vi "Untitled 1.vi"() -> ()   [LabVIEW 2016]
uses:
  DISGradingMachine/MotionPackage/MotionPack/DISActFunc.ctl
panel:
  out "appended array 2":T1[](array[typedef])
  in  "appended array":T1[](array[typedef])
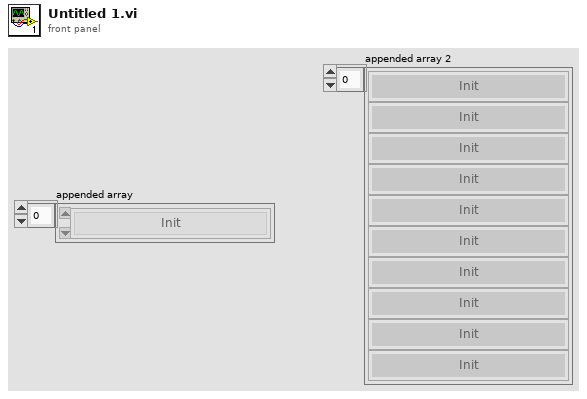
[diagram p1: front panel]
types:
  T1 = typedef "DISActFunc.ctl" = enum16{"Init", "X1 Go To Vibration Station", "X2 Go To DetectPos", "Z1 Go To Upper", "Z2 Go PickingPos(Par_UnitHeight)", "Y1_Go_To_Loose_Unit", "Y2_Go_To_Unit_Wide(Par_UnitWide)", "R Station1", "R Station2", "R Station3", "R Station4", "R Station5", "R Station6", "R Station7", "Vibration On", "Vibration Off", "1_Vacuum_On", "2_Vacuum_On", "3_Vacuum_On", "4_Vacuum_On", "5_Vacuum_On", "6_Vacuum_On", "1_Check_Vacuum", "2_Check_Vacuum", "3_Check_Vacuum", "4_Check_Vacuum", "5_Check_Vacuum", "6_Check_Vacuum", "Vacuum_All_Off", "Vacuum_All_Relief", "Pick6_Vacuum_Relief", "Cylinder_Fix_Unit", "Cylinder_UnFix_Unit", "Level_Probe_Cylinder_Extends", "Level_Probe_Cylinder_Retract", "Vertical_Probe_Cylinder_Extends", "Vertical_Probe_Cylinder_Retract", "Feeder_Inposition_On?"}
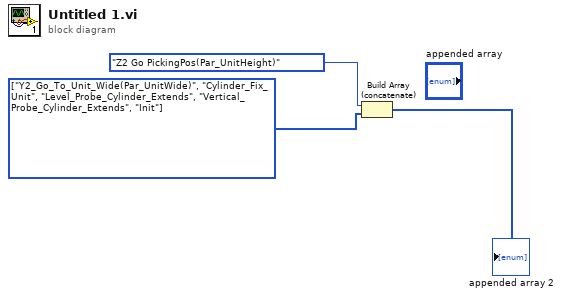
[diagram p0: block diagram]
diagram:
  w3 = T1[] [enum."Y2_Go_To_Unit_Wide(Par_UnitWide)", enum."Cylinder_Fix_Unit", enum."Level_Probe_Cylinder_Extends", enum."Vertical_Probe_Cylinder_Extends", enum."Init"] items=["Init", "X1 Go To Vibration Station", "X2 Go To DetectPos", "Z1 Go To Upper", "Z2 Go PickingPos(Par_UnitHeight)", "Y1_Go_To_Loose_Unit", "Y2_Go_To_Unit_Wide(Par_UnitWide)", "R Station1", "R Station2", "R Station3", "R Station4", "R Station5", "R Station6", "R Station7", "Vibration On", "Vibration Off", "1_Vacuum_On", "2_Vacuum_On", "3_Vacuum_On", "4_Vacuum_On", "5_Vacuum_On", "6_Vacuum_On", "1_Check_Vacuum", "2_Check_Vacuum", "3_Check_Vacuum", "4_Check_Vacuum", "5_Check_Vacuum", "6_Check_Vacuum", "Vacuum_All_Off", "Vacuum_All_Relief", "Pick6_Vacuum_Relief", "Cylinder_Fix_Unit", "Cylinder_UnFix_Unit", "Level_Probe_Cylinder_Extends", "Level_Probe_Cylinder_Retract", "Vertical_Probe_Cylinder_Extends", "Vertical_Probe_Cylinder_Retract", "Feeder_Inposition_On?"]
  n1 = Build Array (concatenate)(DISActFunc."Z2 Go PickingPos(Par_UnitHeight)" ("ActFunc"), w3) -> (→"appended array 2":T1[])
